vi "Catch_screw(stow_side).vi"(6 "向哪校正":T1(ring)=enum."left", 7 "櫃子在哪?":enum16{"前面", "左邊", "右邊"}(ring), 8 "Error In":errorcluster) -> (0 "Error Out":errorcluster, 3 "it2(nut)":string)   [LabVIEW 2019]
uses:
  WSCbot_V3_Toolkit.lvlibp/WSCBOTV3_Toolkit/IO/LowLevel/PulseCounter.ctl
  WSCbot_V3_Toolkit.lvlibp
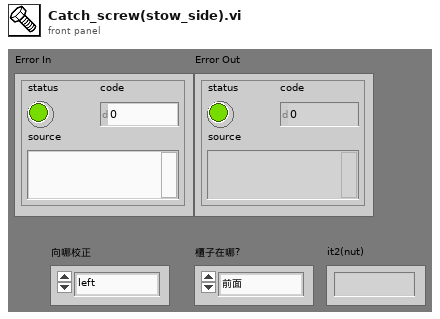
[diagram p1: front panel]
types:
  T1 = enum16{"Right_up", "Right_down", "Left_down", "Left_up", "left", "right", "up", "down"}
  T2 = typedef "WSCbot_V3_Toolkit.lvlibp/PulseCounter.ctl" = enum16{"CH1", "CH2", "CH3", "CH4", "CH5"}
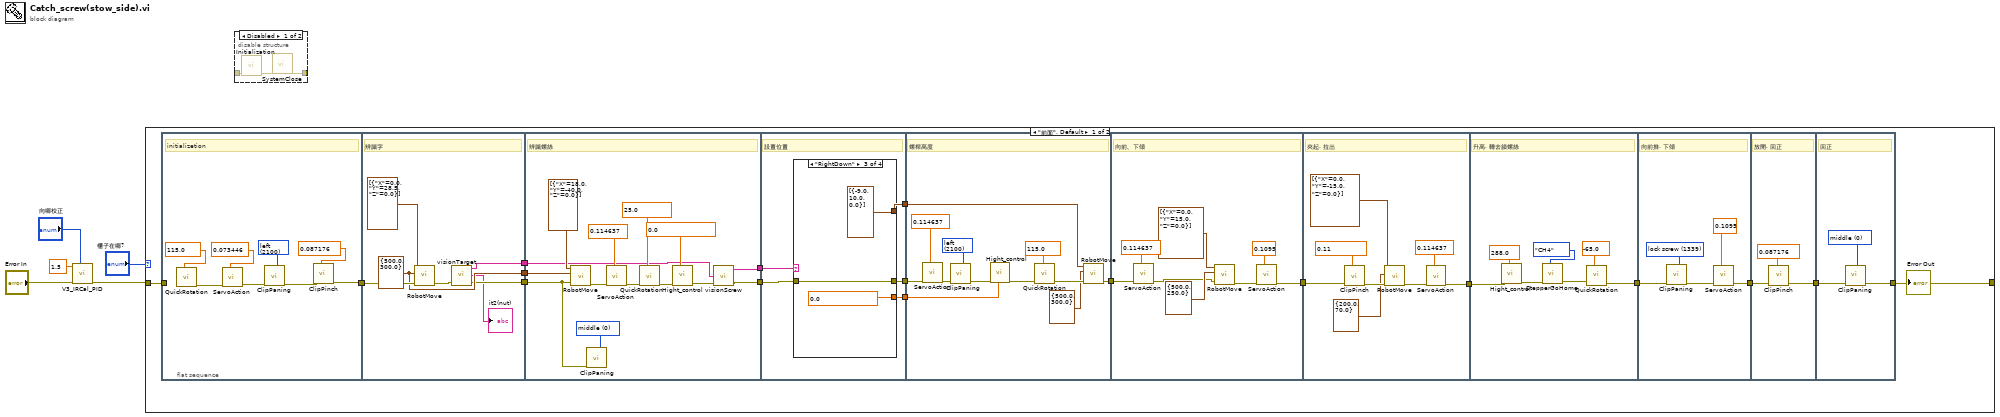
[diagram p0: block diagram]
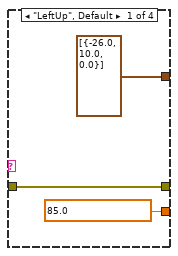
[diagram p2: hidden frame]
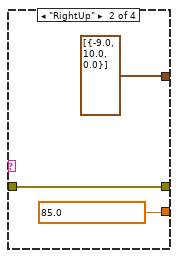
[diagram p3: hidden frame]
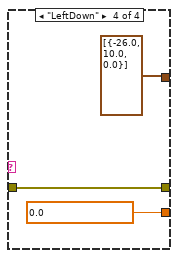
[diagram p4: hidden frame]
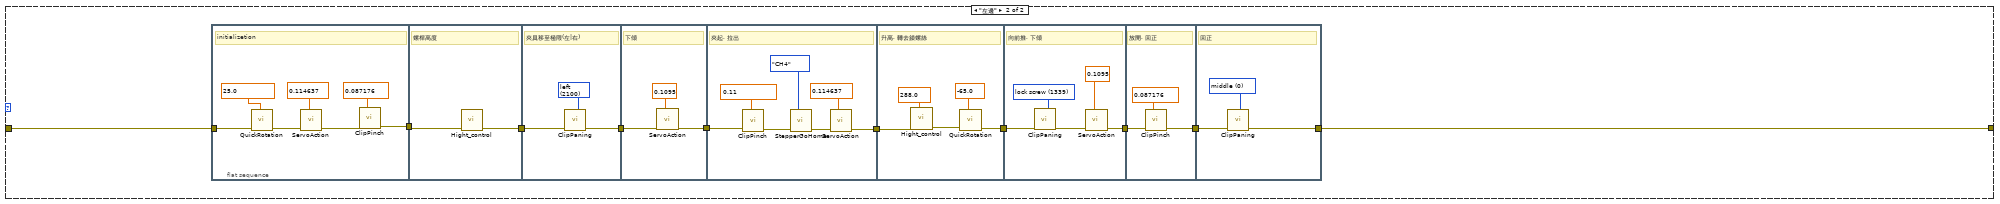
[diagram p5: hidden frame]
diagram:
  n1 = call "V3_IRCal_PID.vi"("Direction"="向哪校正", "Error In"="Error In", "X_distance(V)"=1.5) -> ("Error Out"=w4:errorcluster)  [unwired: 7 in, 1 out]
  n2 = case shown="\"前面\", Default" "櫃子在哪?" {
    tunnel: [w17 w117] -> w6
    tunnel: w4 -> [w18 w116]
    frame "前面", Default {
      n3 = flat-sequence {
        tunnel: [w24] -> w16
        tunnel: w18 -> [_]
        tunnel: w16 -> [w37]
        tunnel: [w36] -> w15
        tunnel: [w35] -> w14
        tunnel: [w33] -> w13
        tunnel: w15 -> [w40]
        tunnel: w14 -> [w45]
        tunnel: w13 -> [w43]
        tunnel: [w39] -> w11
        tunnel: [w41] -> w10
        tunnel: w11 -> [w57]
        tunnel: w10 -> [w56]
        tunnel: [w55] -> w9
        tunnel: [w54] -> w8
        tunnel: [w53] -> w7
        tunnel: [w79] -> w12
        tunnel: w9 -> [w78]
        tunnel: w8 -> [w76]
        tunnel: w7 -> [w73]
        tunnel: [w89] -> w23
        tunnel: w12 -> [w83]
        tunnel: [w95] -> w22
        tunnel: w23 -> [w96]
        tunnel: w22 -> [w102]
        tunnel: [w103] -> w21
        tunnel: w21 -> [w109]
        tunnel: [w105] -> w20
        tunnel: w20 -> [w112]
        tunnel: [w110] -> w19
        tunnel: w19 -> [w114]
        tunnel: [w113] -> w17
        frame #0 {
          w27 = 2100 items=["left"=2100, "right"=-3500, "lock screw"=1339, "middle"=0] ("location")
          w30 = 115.0 items=["Forward"=25.0, "Right"=115.0, "Left"=-65.0] ("螺桿面向")
          w29 = 0.087176 items=["pinch_up"=0.11, "release"=0.087176] ("pinch?")
          w28 = 0.073446 items=["up"=0.1095, "up_up"=0.114637, "down"=0.073446, "back"=0.037435, "back_back"=0.035] ("face_dir")
          # "initializetion"
          n4 = call "QuickRotation.vi"("螺桿面向"=w30) -> ("Error Out"=w31:errorcluster)  [unwired: 10 in]
          n5 = call "ServoAction.vi"("face_dir"=w28, "Error In"=w31) -> ("Error Out"=w25:errorcluster)  [unwired: 9 in]
          n6 = call "ClipPaning.vi"("Error In"=w25, "location"=w27) -> ("Error Out"=w26:errorcluster)  [unwired: 8 in]
          n7 = call "ClipPinch.vi"("pinch?"=w29, "Error In"=w26) -> ("Error Out"=w24:errorcluster)  [unwired: 9 in]
        }
        frame #1 {
          w35 = cluster{dbl, dbl} {500.0, 300.0} ("Speed/ACC")
          # "辨識字"
          n8 = call "RobotMove.vi"("error in (no error)"=w37, "Speed/ACC"=w35, "XYZ"=cluster{"X":dbl, "Y":dbl, "Z":dbl}[] [{"X"=0.0, "Y"=28.5, "Z"=0.0}]) -> ("error out"=w34:errorcluster)  [unwired: 8 in]
          n9 = call "visionTarget.vi"("Error In"=w34) -> ("Error Out"=w33:errorcluster, "it2(nut)"=→"it2(nut)":string, "it1(screw)"=w36:string)  [unwired: 2 in]
        }
        frame #2 {
          w44 = 0 items=["left"=2100, "right"=-3500, "lock screw"=1345, "lock_nut"=1167, "middle"=0] ("location")
          w46 = 0.0 items=["物料櫃第一格"=0.0, "物料櫃第二格"=78.0, "螺帽夾取高度"=128.0, "螺帽瞄準"=250.0, "最高"=288.0] ("螺桿高度")
          w48 = 25.0 items=["Forward"=25.0, "Right"=115.0, "Left"=-65.0] ("螺桿面向")
          w50 = 0.114637 items=["up"=0.1095, "lock_up"=0.111528, "up_up"=0.114637, "down"=0.073446, "back"=0.037435, "back_back"=0.035] ("face_dir")
          # "辨識螺絲"
          n10 = call "RobotMove.vi"("error in (no error)"=w43, "Speed/ACC"=w45, "XYZ"=cluster{"X":dbl, "Y":dbl, "Z":dbl}[] [{"X"=18.0, "Y"=-40.0, "Z"=0.0}]) -> ("error out"=w51:errorcluster)  [unwired: 8 in]
          n11 = call "ClipPaning.vi"("Error In"=w43, "location"=w44) -> ()  [unwired: 8 in, 1 out]
          n12 = call "ServoAction.vi"("face_dir"=w50, "Error In"=w51) -> ("Error Out"=w49:errorcluster)  [unwired: 9 in]
          n13 = call "QuickRotation.vi"("螺桿面向"=w48, "Error In"=w49) -> ("Error Out"=w47:errorcluster)  [unwired: 9 in]
          n14 = call "Hight_control.vi"("螺桿高度"=w46, "Error In"=w47) -> ("Error Out"=w42:errorcluster)  [unwired: 9 in]
          n15 = call "visionScrew.vi"("Error In"=w42, "Aim_Color"=w40) -> ("Error Out"=w41:errorcluster, "Position"=w39:string)  [unwired: 2 in]
        }
        frame #3 {
          # "設置位置"
          n16 = case shown="\"RightDown\"" w57 {
            tunnel: [w58 w61 w66 w67] -> w53
            tunnel: w56 -> [w59 w62 w64 w68]
            tunnel: [cluster{"X":dbl, "Y":dbl, "Z":dbl}[] [{"X"=-26.0, "Y"=10.0, "Z"=0.0}] ("XYZ") cluster{"X":dbl, "Y":dbl, "Z":dbl}[] [{"X"=-9.0, "Y"=10.0, "Z"=0.0}] ("XYZ") cluster{"X":dbl, "Y":dbl, "Z":dbl}[] [{"X"=-9.0, "Y"=10.0, "Z"=0.0}] ("XYZ") cluster{"X":dbl, "Y":dbl, "Z":dbl}[] [{"X"=-26.0, "Y"=10.0, "Z"=0.0}] ("XYZ")] -> w55
            tunnel: [w59 w62 w64 w68] -> w54
            frame "LeftUp", Default {
              w58 = 85.0 items=["物料櫃第一格"=0.0, "物料櫃第二格"=85.0, "螺帽夾取高度"=128.0, "螺帽瞄準"=250.0, "最高"=288.0] ("螺桿高度")
            }
            frame "RightUp" {
              w61 = 85.0 items=["物料櫃第一格"=0.0, "物料櫃第二格"=85.0, "螺帽夾取高度"=128.0, "螺帽瞄準"=250.0, "最高"=288.0] ("螺桿高度")
            }
            frame "RightDown" {
              w66 = 0.0 items=["物料櫃第一格"=0.0, "物料櫃第二格"=78.0, "螺帽夾取高度"=128.0, "螺帽瞄準"=250.0, "最高"=288.0] ("螺桿高度")
            }
            frame "LeftDown" {
              w67 = 0.0 items=["物料櫃第一格"=0.0, "物料櫃第二格"=78.0, "螺帽夾取高度"=128.0, "螺帽瞄準"=250.0, "最高"=288.0] ("螺桿高度")
            }
          }
        }
        frame #4 {
          w74 = 0.114637 items=["up"=0.1095, "lock_up"=0.111528, "up_up"=0.114637, "down"=0.073446, "back"=0.037435, "back_back"=0.035] ("face_dir")
          w81 = 2100 items=["left"=2100, "right"=-3500, "lock screw"=1345, "lock_nut"=1167, "middle"=0] ("location")
          w72 = 115.0 items=["Forward"=25.0, "Right"=115.0, "Left"=-65.0] ("螺桿面向")
          # "螺桿高度"
          n17 = call "ServoAction.vi"("face_dir"=w74, "Error In"=w76) -> ("Error Out"=w75:errorcluster)  [unwired: 9 in]
          n18 = call "ClipPaning.vi"("Error In"=w75, "location"=w81) -> ("Error Out"=w71:errorcluster)  [unwired: 8 in]
          n19 = call "Hight_control.vi"("螺桿高度"=w73, "Error In"=w71) -> ("Error Out"=w70:errorcluster)  [unwired: 9 in]
          n20 = call "QuickRotation.vi"("螺桿面向"=w72, "Error In"=w70) -> ("Error Out"=w80:errorcluster)  [unwired: 9 in]
          n21 = call "RobotMove.vi"("error in (no error)"=w80, "Speed/ACC"=cluster{dbl, dbl} {500.0, 300.0}, "XYZ"=w78) -> ("error out"=w79:errorcluster)  [unwired: 8 in]
        }
        frame #5 {
          w84 = 0.114637 items=["up"=0.1095, "up_up"=0.114637, "down"=0.073446, "back"=0.037435, "back_back"=0.035] ("face_dir")
          w88 = 0.1095 items=["up"=0.1095, "up_up"=0.114637, "down"=0.073446, "back"=0.037435, "back_back"=0.035] ("face_dir")
          # "向前、下傾"
          n22 = call "ServoAction.vi"("face_dir"=w84, "Error In"=w83) -> ("Error Out"=w82:errorcluster)  [unwired: 9 in]
          n23 = call "RobotMove.vi"("error in (no error)"=w82, "Speed/ACC"=cluster{dbl, dbl} {500.0, 250.0}, "XYZ"=cluster{"X":dbl, "Y":dbl, "Z":dbl}[] [{"X"=0.0, "Y"=15.0, "Z"=0.0}]) -> ("error out"=w87:errorcluster)  [unwired: 8 in]
          n24 = call "ServoAction.vi"("face_dir"=w88, "Error In"=w87) -> ("Error Out"=w89:errorcluster)  [unwired: 9 in]
        }
        frame #6 {
          w94 = 0.114637 items=["up"=0.1095, "up_up"=0.114637, "down"=0.073446, "back"=0.037435, "back_back"=0.035] ("face_dir")
          w97 = 0.11 items=["pinch_up"=0.11, "release"=0.087176] ("pinch?")
          # "夾起, 拉出"
          n25 = call "ClipPinch.vi"("pinch?"=w97, "Error In"=w96) -> ("Error Out"=w93:errorcluster)  [unwired: 9 in]
          n26 = call "RobotMove.vi"("error in (no error)"=w93, "Speed/ACC"=cluster{dbl, dbl} {200.0, 70.0}, "XYZ"=cluster{"X":dbl, "Y":dbl, "Z":dbl}[] [{"X"=0.0, "Y"=-15.0, "Z"=0.0}]) -> ("error out"=w92:errorcluster)  [unwired: 8 in]
          n27 = call "ServoAction.vi"("face_dir"=w94, "Error In"=w92) -> ("Error Out"=w95:errorcluster)  [unwired: 9 in]
        }
        frame #7 {
          w101 = 288.0 items=["物料櫃第一格"=0.0, "物料櫃第二格"=78.0, "螺帽夾取高度"=128.0, "螺帽瞄準"=250.0, "最高"=288.0] ("螺桿高度")
          w104 = -65.0 items=["Forward"=25.0, "Right"=115.0, "Left"=-65.0] ("螺桿面向")
          # "升高, 轉去鎖螺絲"
          n28 = call "Hight_control.vi"("螺桿高度"=w101, "Error In"=w102) -> ("Error Out"=w99:errorcluster)  [unwired: 9 in]
          n29 = call "StepperGoHome.vi"("PulseCounterChanel"=PulseCounter."CH4", "Error In"=w99) -> ("Error Out"=w98:errorcluster)  [unwired: 7 in, 2 out]
          n30 = call "QuickRotation.vi"("螺桿面向"=w104, "Error In"=w98) -> ("Error Out"=w103:errorcluster)  [unwired: 9 in]
        }
        frame #8 {
          w106 = 0.1095 items=["up"=0.1095, "up_up"=0.114637, "down"=0.073446, "back"=0.037435, "back_back"=0.035] ("face_dir")
          w108 = 1339 items=["left"=2100, "right"=-3500, "lock screw"=1339, "middle"=0] ("location")
          # "向前推, 下傾"
          n31 = call "ClipPaning.vi"("Error In"=w109, "location"=w108) -> ("Error Out"=w107:errorcluster)  [unwired: 8 in]
          n32 = call "ServoAction.vi"("face_dir"=w106, "Error In"=w107) -> ("Error Out"=w105:errorcluster)  [unwired: 9 in]
        }
        frame #9 {
          w111 = 0.087176 items=["pinch_up"=0.11, "release"=0.087176] ("pinch?")
          # "放開, 回正"
          n33 = call "ClipPinch.vi"("pinch?"=w111, "Error In"=w112) -> ("Error Out"=w110:errorcluster)  [unwired: 9 in]
        }
        frame #10 {
          w115 = 0 items=["left"=2100, "right"=-3500, "lock screw"=1339, "middle"=0] ("location")
          # "回正"
          n34 = call "ClipPaning.vi"("Error In"=w114, "location"=w115) -> ("Error Out"=w113:errorcluster)  [unwired: 8 in]
        }
      }
    }
    frame "左邊" {
      n35 = flat-sequence {
        tunnel: [w129] -> w125
        tunnel: w116 -> [w127]
        tunnel: w125 -> [w134]
        tunnel: [w133] -> w124
        tunnel: [w137] -> w123
        tunnel: w124 -> [w135]
        tunnel: w123 -> [w139]
        tunnel: [w140] -> w122
        tunnel: [w142] -> w121
        tunnel: w122 -> [w144]
        tunnel: w121 -> [w150]
        tunnel: [w151] -> w120
        tunnel: w120 -> [w157]
        tunnel: [w153] -> w119
        tunnel: w119 -> [w160]
        tunnel: [w158] -> w118
        tunnel: w118 -> [w162]
        tunnel: [w161] -> w117
        frame #0 {
          w126 = 25.0 items=["Forward"=25.0, "Right"=115.0, "Left"=-65.0] ("螺桿面向")
          w131 = 0.087176 items=["pinch_up"=0.11, "release"=0.087176] ("pinch?")
          w132 = 0.114637 items=["up"=0.1095, "up_up"=0.114637, "down"=0.073446, "back"=0.037435, "back_back"=0.035] ("face_dir")
          # "initializetion"
          n36 = call "QuickRotation.vi"("螺桿面向"=w126, "Error In"=w127) -> ("Error Out"=w128:errorcluster)  [unwired: 9 in]
          n37 = call "ServoAction.vi"("face_dir"=w132, "Error In"=w128) -> ("Error Out"=w130:errorcluster)  [unwired: 9 in]
          n38 = call "ClipPinch.vi"("pinch?"=w131, "Error In"=w130) -> ("Error Out"=w129:errorcluster)  [unwired: 9 in]
        }
        frame #1 {
          # "螺桿高度"
          n39 = call "Hight_control.vi"("Error In"=w134) -> ("Error Out"=w133:errorcluster)  [unwired: 10 in]
        }
        frame #2 {
          w136 = 2100 items=["left"=2100, "right"=-3500, "lock screw"=1339, "middle"=0] ("location")
          # "夾具移至極限(左|右)"
          n40 = call "ClipPaning.vi"("Error In"=w135, "location"=w136) -> ("Error Out"=w137:errorcluster)  [unwired: 8 in]
        }
        frame #3 {
          w138 = 0.1095 items=["up"=0.1095, "up_up"=0.114637, "down"=0.073446, "back"=0.037435, "back_back"=0.035] ("face_dir")
          # "下傾"
          n41 = call "ServoAction.vi"("face_dir"=w138, "Error In"=w139) -> ("Error Out"=w140:errorcluster)  [unwired: 9 in]
        }
        frame #4 {
          w141 = 0.114637 items=["up"=0.1095, "up_up"=0.114637, "down"=0.073446, "back"=0.037435, "back_back"=0.035] ("face_dir")
          w147 = 0.11 items=["pinch_up"=0.11, "release"=0.087176] ("pinch?")
          # "夾起, 拉出"
          n42 = call "ClipPinch.vi"("pinch?"=w147, "Error In"=w144) -> ("Error Out"=w146:errorcluster)  [unwired: 9 in]
          n43 = call "StepperGoHome.vi"("PulseCounterChanel"=PulseCounter."CH4", "Error In"=w146) -> ("Error Out"=w143:errorcluster)  [unwired: 7 in, 2 out]
          n44 = call "ServoAction.vi"("face_dir"=w141, "Error In"=w143) -> ("Error Out"=w142:errorcluster)  [unwired: 9 in]
        }
        frame #5 {
          w148 = 288.0 items=["物料櫃第一格"=0.0, "物料櫃第二格"=78.0, "螺帽夾取高度"=128.0, "螺帽瞄準"=250.0, "最高"=288.0] ("螺桿高度")
          w152 = -65.0 items=["Forward"=25.0, "Right"=115.0, "Left"=-65.0] ("螺桿面向")
          # "升高, 轉去鎖螺絲"
          n45 = call "Hight_control.vi"("螺桿高度"=w148, "Error In"=w150) -> ("Error Out"=w149:errorcluster)  [unwired: 9 in]
          n46 = call "QuickRotation.vi"("螺桿面向"=w152, "Error In"=w149) -> ("Error Out"=w151:errorcluster)  [unwired: 9 in]
        }
        frame #6 {
          w154 = 0.1095 items=["up"=0.1095, "up_up"=0.114637, "down"=0.073446, "back"=0.037435, "back_back"=0.035] ("face_dir")
          w156 = 1339 items=["left"=2100, "right"=-3500, "lock screw"=1339, "middle"=0] ("location")
          # "向前推, 下傾"
          n47 = call "ClipPaning.vi"("Error In"=w157, "location"=w156) -> ("Error Out"=w155:errorcluster)  [unwired: 8 in]
          n48 = call "ServoAction.vi"("face_dir"=w154, "Error In"=w155) -> ("Error Out"=w153:errorcluster)  [unwired: 9 in]
        }
        frame #7 {
          w159 = 0.087176 items=["pinch_up"=0.11, "release"=0.087176] ("pinch?")
          # "放開, 回正"
          n49 = call "ClipPinch.vi"("pinch?"=w159, "Error In"=w160) -> ("Error Out"=w158:errorcluster)  [unwired: 9 in]
        }
        frame #8 {
          w163 = 0 items=["left"=2100, "right"=-3500, "lock screw"=1339, "middle"=0] ("location")
          # "回正"
          n50 = call "ClipPaning.vi"("Error In"=w162, "location"=w163) -> ("Error Out"=w161:errorcluster)  [unwired: 8 in]
        }
      }
    }
  }
  "Error Out" <- w6
  n51 = disable-structure shown="Disabled" {
    disable-tunnel: [w165 _] -> _
    disable-tunnel: _ -> [w164 _]
    frame Disabled {
      n52 = call "Initialization.vi"("Error In"=w164) -> ("Error Out"=w165:errorcluster)  [unwired: 10 in]
      n53 = call "SystemClose.vi"() -> ()  [unwired: 3 in, 1 out]
    }
    frame Enabled {
    }
  }
